vi "субприборо кластера.vi"() -> (3 "Cluster":T1)   [LabVIEW 2017]
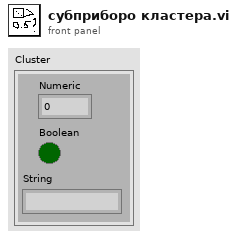
[diagram p1: front panel]
types:
  T1 = cluster{"Numeric":dbl, "Boolean":bool, "String":string}
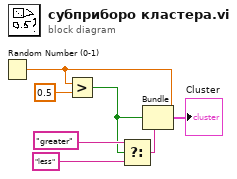
[diagram p0: block diagram]
diagram:
  n1 = Random Number (0-1)() -> (number: 0 to 1=w4:dbl)
  n2 = Greater?(x=w4, y=0.5) -> (0:w2:bool)
  n3 = Select(t="greater", s=w2, f="less") -> (s? t:f=w3:string)
  n4 = Bundle("number: 0 to 1"=w4, w2, w3) -> (→"Cluster":cluster{"number: 0 to 1":dbl, bool, string})  [unwired: 1 in]
